vi "Query System Date.vi"(8 "error in (no error)":errorcluster, 11 "VISA resource name":refnum<visa-resource-name>) -> (0 "error out":errorcluster, 1 "Month":i32, 2 "Year":i32, 3 "VISA resource name out":refnum<visa-resource-name>, 4 "Day":i32)   [LabVIEW 2015, in "Rohde&Schwarz CMXP Base.lvlib"]
doc: "Queries the UTC date of the operating system calendar.\n\nAttribute:\n-\n\nRemote-control command:\nSYSTem:DATE[:UTC]"
uses:
  <instrlib>/Rohde&Schwarz CMXP Base/Rohde&Schwarz CMXP Base.lvlib
  <instrlib>/Rohde&Schwarz CMXP Base/Private/rsidr_core.llb/rsidr_core.lvlib
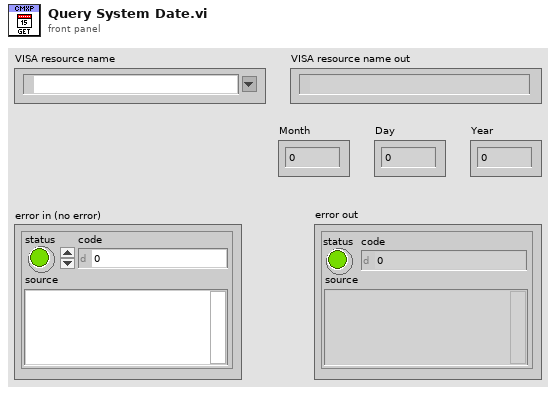
[diagram p1: front panel]
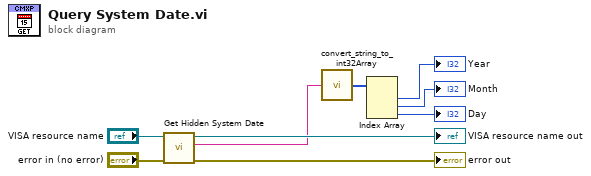
[diagram p0: block diagram]
diagram:
  n1 = call "Get Hidden System Date"("error in (no error)"="error in (no error)", "instrument handle"="VISA resource name") -> ("error out"=→"error out":errorcluster, "Hidden System Date"=w3:string, "instrument handle out"=→"VISA resource name out":refnum<visa-resource-name>)  [unwired: 7 in]
  n2 = call <instrlib>:"convert_string_to_int32Array.vi"("string in"=w3) -> ("int32 array out"=w7:i32[])  [unwired: 3 in, 1 out]
  n3 = Index Array(array=w7) -> (element #1=→"Year":i32, element #2=→"Month":i32, element #3=→"Day":i32)  [unwired: 3 in]
